vi "create standard file path.vi"(7 "name or relative path":string, 8 "error in (no error)":errorcluster) -> (0 "error out":errorcluster, 4 "appended path":path)   [LabVIEW 2012]
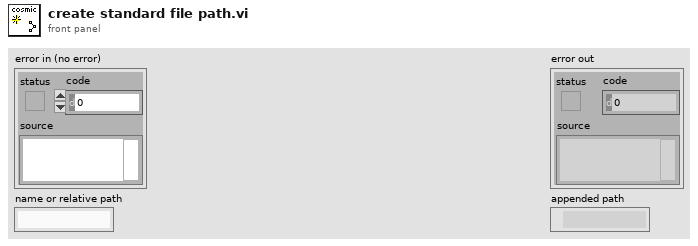
[diagram p1: front panel]
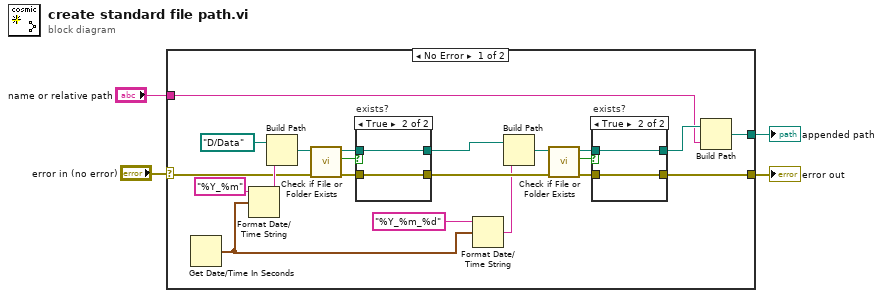
[diagram p0: block diagram]
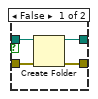
[diagram p2: hidden frame]
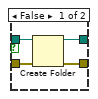
[diagram p3: hidden frame]
diagram:
  n1 = case shown="No Error" "error in (no error)" {
    selector: "error in (no error)" -> [w8 w38]
    tunnel: [w9 w38] -> w3
    tunnel: "name or relative path" -> [w6 _]
    tunnel: [w5 _] -> w1
    frame No Error {
      n2 = Get Date/Time In Seconds() -> (seconds since 1Jan1904=w24:timestamp)
      n3 = Format Date/Time String(time format string (%c)="%Y_%m", seconds (now)=w24) -> (date/time string=w10:string)  [unwired: 1 in]
      n4 = Build Path(base path=path "D:/Data", name or relative path=w10) -> (appended path=w12:path)
      n5 = call <vilib>:"Check if File or Folder Exists.vi"("error in (no error)"=w8, "path"=w12) -> ("error out"=w15:errorcluster, "file or folder exists?"=w13:bool, "dup path"=w14:path)  [unwired: 7 in]
      n6 = case "exists?" shown="True" w13 {
        tunnel: w14 -> [w34 w36]
        tunnel: w15 -> [w35 w37]
        tunnel: [w33 w36] -> w23
        tunnel: [w32 w37] -> w22
        frame False {
          n7 = Create Folder(path (use dialog)=w34, error in=w35) -> (created path=w33:path, error out=w32:errorcluster)  [unwired: 1 in, 1 out]
        }
        frame True {
        }
      }
      n8 = Format Date/Time String(time format string (%c)="%Y_%m_%d", seconds (now)=w24) -> (date/time string=w20:string)  [unwired: 1 in]
      n9 = Build Path(base path=w23, name or relative path=w20) -> (appended path=w16:path)
      n10 = call <vilib>:"Check if File or Folder Exists.vi"("error in (no error)"=w22, "path"=w16) -> ("error out"=w19:errorcluster, "file or folder exists?"=w17:bool, "dup path"=w18:path)  [unwired: 7 in]
      n11 = case "exists?" shown="True" w17 {
        tunnel: w18 -> [w28 w30]
        tunnel: w19 -> [w29 w31]
        tunnel: [w27 w30] -> w25
        tunnel: [w26 w31] -> w9
        frame False {
          n12 = Create Folder(path (use dialog)=w28, error in=w29) -> (created path=w27:path, error out=w26:errorcluster)  [unwired: 1 in, 1 out]
        }
        frame True {
        }
      }
      n13 = Build Path(base path=w25, name or relative path=w6) -> (appended path=w5:path)
    }
    frame Error {
    }
  }
  "error out" <- w3
  "appended path" <- w1
